vi "Init LCD.vi"(8 "error in (no error)":errorcluster, 10 "VISA resource name in":refnum<visa-resource-name>, 11 "LCD-I2C in":refnum<class "LCD-I2C.lvclass">) -> (0 "error out":errorcluster, 2 "VISA resource name":refnum<visa-resource-name>, 3 "LCD-I2C out":refnum<class "LCD-I2C.lvclass">)   [LabVIEW 2023, in "CTI-Visa-DeviceLib.lvlib" / "LCD-I2C.lvclass"]
uses:
  LCD-I2C.lvclass
  Display Function.ctl
  Bus Mode.ctl
  Lines.ctl
  Glyph Size.ctl
  Display Control.ctl
  Display Mode.ctl
  Entry Shift.ctl
  Glyph Entry.ctl
  LCD-I2C.lvclass/LCD-I2C.ctl
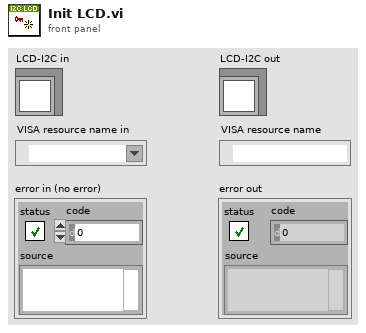
[diagram p1: front panel]
types:
  T1 = typedef "CTI-Visa-DeviceLib.lvlib/LCD-I2C.lvclass/Display Mode.ctl" = cluster{"Entry Shift":T2, "Glyph Entry":T3}
  T2 = typedef "CTI-Visa-DeviceLib.lvlib/LCD-I2C.lvclass/Entry Shift.ctl" = enum8{"Decrement", "Increment"}
  T3 = typedef "CTI-Visa-DeviceLib.lvlib/LCD-I2C.lvclass/Glyph Entry.ctl" = enum8{"Right", "Left"}
  T4 = typedef "CTI-Visa-DeviceLib.lvlib/LCD-I2C.lvclass/Display Control.ctl" = cluster{"Blink On":bool, "Cursor On":bool, "Display On":bool}
  T5 = typedef "CTI-Visa-DeviceLib.lvlib/LCD-I2C.lvclass/Glyph Size.ctl" = enum8{"5x8", "5x10"}
  T6 = typedef "CTI-Visa-DeviceLib.lvlib/LCD-I2C.lvclass/Bus Mode.ctl" = enum8{"4 Bit", "8 Bit"}
  T7 = typedef "CTI-Visa-DeviceLib.lvlib/LCD-I2C.lvclass/Lines.ctl" = enum8{"Single", "Multiline"}
  T8 = typedef "CTI-Visa-DeviceLib.lvlib/LCD-I2C.lvclass/Display Function.ctl" = cluster{"Bus Mode":T6, "Lines":T7, "Glyph Size":T5}
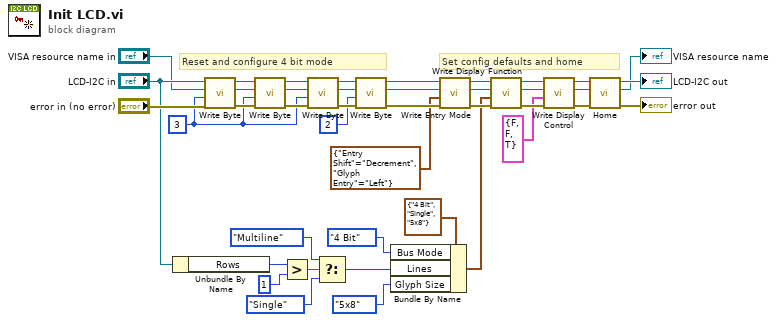
[diagram p0: block diagram]
diagram:
  w16 = u8 3 ("Value")
  # "Set config defaults and home"
  # "Reset and configure 4 bit mode"
  n1 = Unbundle By Name("LCD-I2C in") -> ("Rows"=w38:u8)
  n2 = call "Write Byte.vi"("error in (no error)"="error in (no error)", "Value"=w16, "VISA resource name in"="VISA resource name in", "LCD-I2C in"="LCD-I2C in") -> ("error out"=w20:errorcluster, "VISA resource name"=w18:refnum<visa-resource-name>, "LCD-I2C out"=w22:refnum<class "LCD-I2C.lvclass">)  [unwired: 5 in]
  n3 = call "Write Byte.vi"("error in (no error)"=w20, "Value"=w16, "VISA resource name in"=w18, "LCD-I2C in"=w22) -> ("error out"=w19:errorcluster, "VISA resource name"=w17:refnum<visa-resource-name>, "LCD-I2C out"=w21:refnum<class "LCD-I2C.lvclass">)  [unwired: 5 in]
  n4 = Greater?(x=w38, y=u8 1) -> (0:w36:bool)
  n5 = call "Write Byte.vi"("error in (no error)"=w19, "Value"=w16, "VISA resource name in"=w17, "LCD-I2C in"=w21) -> ("error out"=w15:errorcluster, "VISA resource name"=w13:refnum<visa-resource-name>, "LCD-I2C out"=w14:refnum<class "LCD-I2C.lvclass">)  [unwired: 5 in]
  n6 = Select(t=Lines."Multiline" ("Lines"), s=w36, f=Lines."Single" ("Lines")) -> (s? t:f=w32:T7)
  n7 = call "Write Byte.vi"("error in (no error)"=w15, "Value"=u8 2, "VISA resource name in"=w13, "LCD-I2C in"=w14) -> ("error out"=w40:errorcluster, "VISA resource name"=w10:refnum<visa-resource-name>, "LCD-I2C out"=w11:refnum<class "LCD-I2C.lvclass">)  [unwired: 5 in]
  n8 = Bundle By Name(cluster=T8 {"Bus Mode"=enum."4 Bit", "Lines"=enum."Single", "Glyph Size"=enum."5x8"} ("Display Function"), "Bus Mode"=Bus_Mode."4 Bit", "Lines"=w32, "Glyph Size"=Glyph_Size."5x8") -> (w6:T8)
  n9 = call "Write Entry Mode.vi"("error in (no error)"=w40, "Display Mode"=T1 {"Entry Shift"=enum."Decrement", "Glyph Entry"=enum."Left"}, "VISA resource name in"=w10, "LCD-I2C in"=w11) -> ("error out"=w9:errorcluster, "VISA resource name"=w7:refnum<visa-resource-name>, "LCD-I2C out"=w8:refnum<class "LCD-I2C.lvclass">)  [unwired: 5 in]
  n10 = call "Write Display Function.vi"("error in (no error)"=w9, "Display Function"=w6, "VISA resource name in"=w7, "LCD-I2C in"=w8) -> ("error out"=w41:errorcluster, "VISA resource name"=w1:refnum<visa-resource-name>, "LCD-I2C out"=w5:refnum<class "LCD-I2C.lvclass">)  [unwired: 5 in]
  n11 = call "Write Display Control.vi"("error in (no error)"=w41, "Display Control"=T4 {"Blink On"=FALSE, "Cursor On"=FALSE, "Display On"=TRUE}, "VISA resource name in"=w1, "LCD-I2C in"=w5) -> ("error out"=w4:errorcluster, "VISA resource name"=w2:refnum<visa-resource-name>, "LCD-I2C out"=w3:refnum<class "LCD-I2C.lvclass">)  [unwired: 5 in]
  n12 = call "Home.vi"("error in (no error)"=w4, "VISA resource name in"=w2, "LCD-I2C in"=w3) -> ("error out"=→"error out":errorcluster, "VISA resource name"=→"VISA resource name":refnum<visa-resource-name>, "LCD-I2C out"=→"LCD-I2C out":refnum<class "LCD-I2C.lvclass">)  [unwired: 6 in]
